vi "tlc_Record.vi"(8 "error in (no error)":errorcluster, 10 "Cue":T1 {"Channels"."Intensität" min=0.0 max=100.0 step=1.0 format="%#.0f"}) -> (0 "error out":errorcluster)   [LabVIEW 2010]
uses:
  Controls/tlc_Cue_Information.ctl
  Controls/channel.ctl
  Controls/tlc_User Interface Data Type.ctl
  Modules/Cue/tlc_Cue_Information Command.ctl
panel:
  # "Input"
  # "Output"
  # "This is the cue that is to be added to the cue list.  Once tlc_Cue_Information.ctl has been completed, this control will be filled in."
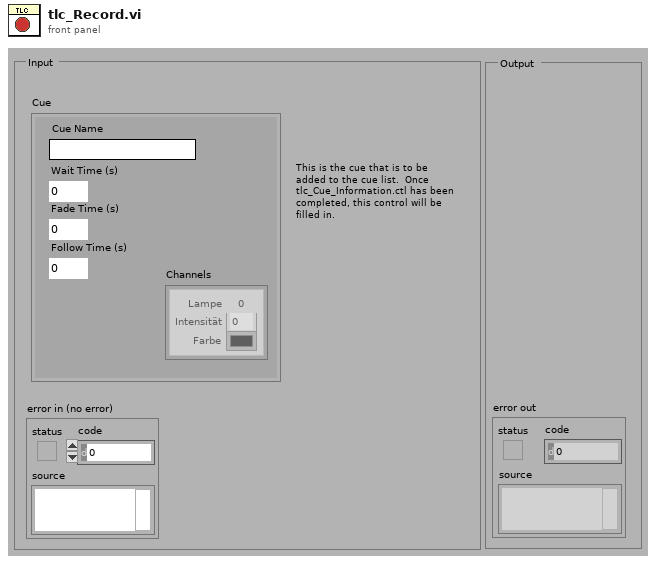
[diagram p1: front panel]
types:
  T1 = typedef "tlc_Cue_Information.ctl" = cluster{"Cue Name":string, "Wait Time (s)":u32, "Fade Time (s)":u32, "Follow Time (s)":u32, "Channels":T2[][]}
  T2 = typedef "channel.ctl" = cluster{"Intensität":dbl, " Farbe":u32, "Channel":i32}
  T3 = typedef "tlc_User Interface Data Type.ctl" = enum16{"Initialize", "Initialize Front Panel", "Update Front Panel Channels", "Select Cue in Cue List", "Enable/Disable Front Panel Controls", "Update Cue List", "Stop"}
  T4 = typedef "tlc_Cue_Information Command.ctl" = enum16{"Add Cue", "Get Cue Values", "Set Cue Values", "Get Number of Cues", "Initialize", "Get Empty Cue"}
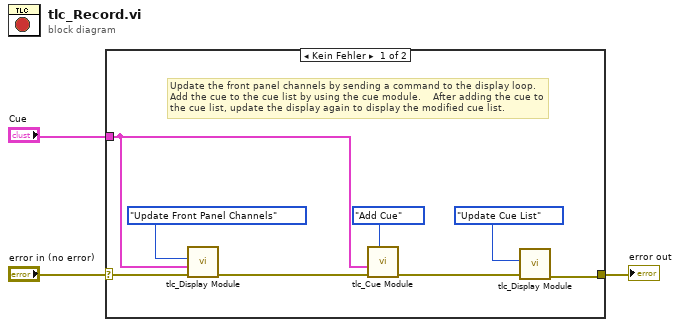
[diagram p0: block diagram]
diagram:
  n1 = case shown="Kein Fehler" "error in (no error)" {
    selector: "error in (no error)" -> [w11 w12]
    tunnel: "Cue" -> [w7 _]
    tunnel: [w5 w12] -> w2
    frame No Error {
      # "Update the front panel channels by sending a command to the display loop.  Add the cue to the cue list by using the cue module.    After adding the cue to the cue list, update the display again to display the modified cue list."
      n2 = call "tlc_Display Module.vi"("error in (no error)"=w11, "Data"=w7, "Data Type"=tlc_User_Interface_Data_Type."Update Front Panel Channels") -> ("error out"=w9:errorcluster)  [unwired: 8 in]
      n3 = call "tlc_Cue Module.vi"("Command"=tlc_Cue_Information_Command."Add Cue", "error in (no error)"=w9, "Cue Input"=w7) -> ("error out"=w6:errorcluster)  [unwired: 5 in, 2 out]
      n4 = call "tlc_Display Module.vi"("error in (no error)"=w6, "Data Type"=tlc_User_Interface_Data_Type."Update Cue List") -> ("error out"=w5:errorcluster)  [unwired: 9 in]
    }
    frame Error {
    }
  }
  "error out" <- w2
